vi "JSON Value to Variant.vi"(8 "error in (no error)":errorcluster, 11 "JSON Value in":refnum<class "JSON Value.lvclass">) -> (0 "error out":errorcluster, 3 "Variant out":variant)   [LabVIEW 2016, in "JSON Variant Support.lvclass"]
uses:
  JSON Variant Support.lvclass
  JSON Value/JSON Value.lvclass
  JSON Value/Read Value/Read value (Numeric).vi
  JSON Value/Read Value/Read value (Boolean).vi
  JSON Value/Read Value/Read value (String).vi
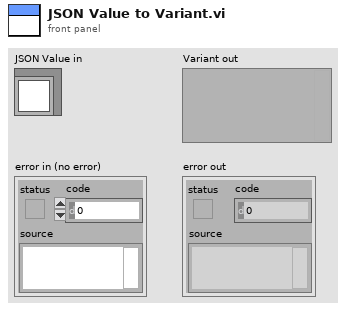
[diagram p1: front panel]
types:
  T1 = typedef "JSON Value.lvclass/JSON Types.ctl" = enum16{"String", "Numeric", "Boolean", "NULL", "Object", "Array"}
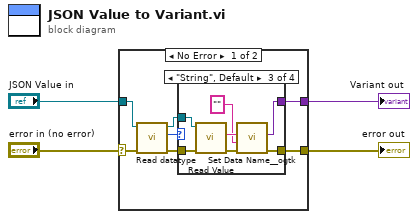
[diagram p0: block diagram]
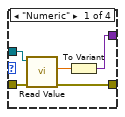
[diagram p2: hidden frame]
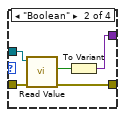
[diagram p3: hidden frame]
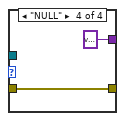
[diagram p4: hidden frame]
diagram:
  n1 = case shown="No Error" "error in (no error)" {
    selector: "error in (no error)" -> [w10 w31]
    tunnel: [w5 w31] -> w3
    tunnel: "JSON Value in" -> [w11 _]
    tunnel: [w6 _] -> w1
    frame No Error {
      n2 = call "Read datatype.vi"("error in (no error)"=w10, "JSON Value in"=w11) -> ("error out"=w7:errorcluster, "datatype"=w9:T1, "JSON Value out"=w8:refnum<class "JSON Value.lvclass">)  [unwired: 7 in]
      n3 = case shown="\"String\", Default" w9 {
        tunnel: w8 -> [w16 w21 w28 _]
        tunnel: w7 -> [w15 w20 w27 w30]
        tunnel: [w13 w18 w26 variant ("Variant")] -> w6
        tunnel: [w12 w17 w23 w30] -> w5
        frame "Numeric" {
          n4 = call-poly "Read Value.vi"("error in (no error)"=w15, "JSON Numeric in"=w16) -> ("error out"=w12:errorcluster, "value"=w14:dbl)  [unwired: 7 in, 1 out]
          n5 = To Variant(anything=w14) -> (Variant=w13:variant)
        }
        frame "Boolean" {
          n6 = call-poly "Read Value.vi"("error in (no error)"=w20, "JSON Boolean in"=w21) -> ("error out"=w17:errorcluster, "value"=w19:bool)  [unwired: 7 in, 1 out]
          n7 = To Variant(anything=w19) -> (Variant=w18:variant)
        }
        frame "String", Default {
          n8 = call-poly "Read Value.vi"("error in (no error)"=w27, "JSON String in"=w28) -> ("error out"=w24:errorcluster, "value"=w25:string)  [unwired: 7 in, 1 out]
          n9 = call <userlib>:"Set Data Name__ogtk.vi"("error in (no error)"=w24, "Data Name"="", "Data"=w25) -> ("error out"=w23:errorcluster, "Renamed Data"=w26:variant)  [unwired: 7 in]
        }
        frame "NULL" {
        }
      }
    }
    frame Error {
    }
  }
  "error out" <- w3
  "Variant out" <- w1
